vi "NIIE_Draw Point.vi"(4 "Edge Color":u32(colorbox), 6 "Fill Color":u32(colorbox), 8 "Error":errorcluster, 9 "Current Color (T)":u32(colorbox)=16777216, 11 "Point(x,y)":cluster{"x":i16, "y":i16}) -> (0 "Error Out":errorcluster, 3 "New Picture Out":picture, 5 "Current Line Color Out":u32(colorbox))   [LabVIEW 2021]
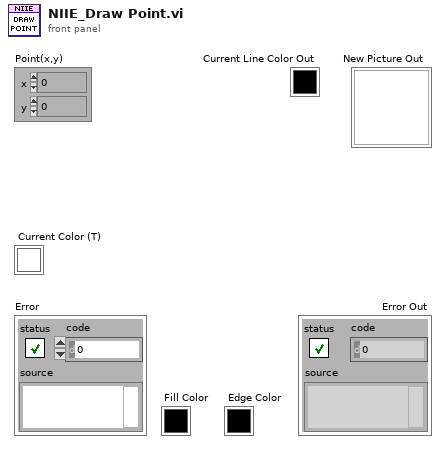
[diagram p1: front panel]
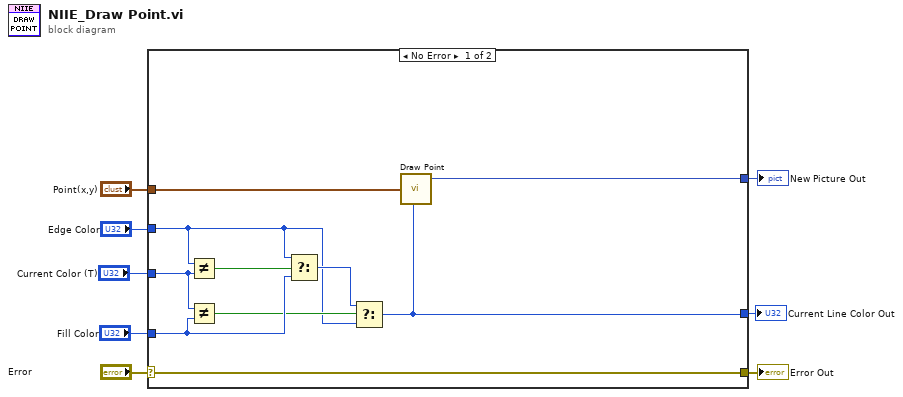
[diagram p0: block diagram]
diagram:
  n1 = case shown="No Error" "Error" {
    selector: "Error" -> [w18 w19]
    tunnel: [w18 w19] -> w7
    tunnel: [w17 _] -> w6
    tunnel: "Point(x,y)" -> [w16 _]
    tunnel: "Edge Color" -> [w10 _]
    tunnel: "Current Color (T)" -> [w15 _]
    tunnel: "Fill Color" -> [w14 _]
    tunnel: [w9 _] -> w1
    frame No Error {
      n2 = Not Equal?(x=w10, y=w15) -> (x != y?=w12:bool)
      n3 = Not Equal?(x=w15, y=w14) -> (x != y?=w13:bool)
      n4 = Select(t=w10, s=w12, f=w14) -> (s? t:f=w11:u32)
      n5 = Select(t=w11, s=w13, f=w10) -> (s? t:f=w9:u32)
      n6 = call <vilib>:"Draw Point.vi"("point(x,y)"=w16, "color(black)"=w9) -> ("new picture"=w17:picture)  [unwired: 2 in, 5 out]
    }
    frame Error {
    }
  }
  "Error Out" <- w7
  "New Picture Out" <- w6
  "Current Line Color Out" <- w1
